vi "DigitalIORead.vi"(0 "error in":errorcluster, 2 "Component":T1, 3 "node":string) -> (1 "error out":errorcluster, 4 "Digital IO State":cluster{"state":i8, "is input only":bool})   [LabVIEW 2015]
doc: "Read a digital output"
uses:
  ROS/Code/SubVIs/DigitalIOComponents.ctl
  ROS/Code/Console/Servers/ServerSubs/TopicDef.ctl
  ROS/Code/SubVIs/_ROSDirection.ctl
panel:
  out "Reply":string
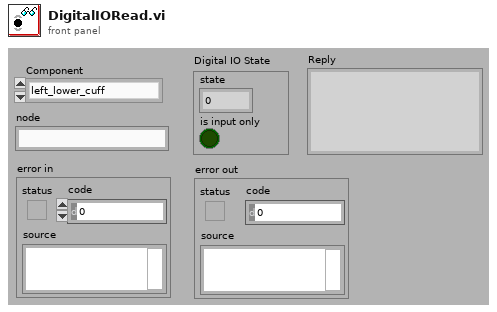
[diagram p1: front panel]
types:
  T1 = typedef "DigitalIOComponents.ctl" = enum16{"left_lower_cuff", "right_lower_cuff", "left_lower_button", "right_lower_button", "left_upper_button", "right_upper_button", "left_shoulder_button", "right_shoulder_button"}
  T2 = typedef "TopicDef.ctl" = cluster{"Topic":string, "Type":string, "Action":T3, "Update (ms)":u16, "queue size":u16}
  T3 = typedef "_ROSDirection.ctl" = enum16{"Node", "Publisher", "Subscriber", "ServiceClient", "ServiceProvider"}
  T4 = typedef "_ROSControl.ctl" = cluster{"topic port":u16, "Node":string, "topic":string, "type":string, "node port":u16, "error ":errorcluster, "Direction":T3, "Update (ms)":u16, "FIFO size":u16}
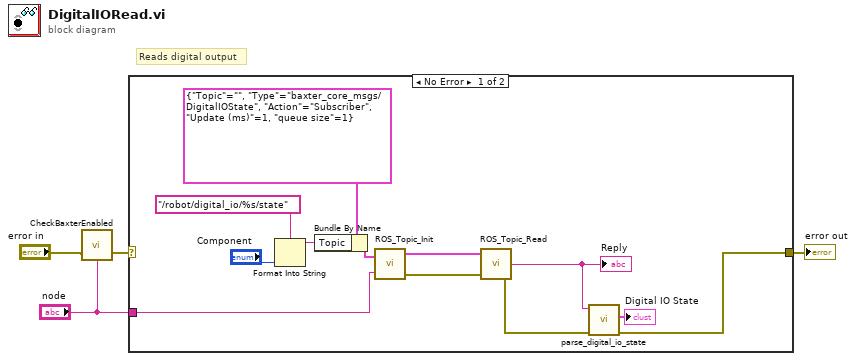
[diagram p0: block diagram]
diagram:
  # "Reads digital output"
  n1 = call "CheckBaxterEnabled.vi"("error in"="error in", "node"="node") -> ("error out"=w2:errorcluster)  [unwired: 2 in]
  n2 = case shown="No Error" w2 {
    selector: w2 -> [_ w17]
    tunnel: [w5 w17] -> w4
    tunnel: "node" -> [w8 _]
    frame No Error {
      n3 = Format Into String(format string="/robot/digital_io/%s/state" ("topic"), "Component") -> (resulting string=w11:string)  [unwired: 2 in, 1 out]
      n4 = Bundle By Name(cluster=T2 {"Topic"="", "Type"="baxter_core_msgs/DigitalIOState", "Action"=enum."Subscriber", "Update (ms)"=1, "queue size"=1} ("Definitions"), "Topic"=w11) -> (w10:T2)
      n5 = call "ROS_Topic_Init.vi"("Definitions"=w10, "node"=w8) -> ("ROS out"=w16:T4, "error out"=w6:errorcluster)  [unwired: 1 in]
      n6 = call "ROS_Topic_Read.vi"("error in (no error)"=w6, "ROS in"=w16) -> ("error out"=w7:errorcluster, "Reply"=w15:string)  [unwired: 1 in, 1 out]
      "Reply" <- w15
      n7 = call "parse_digital_io_state.vi"("error in"=w7, "msg in"=w15) -> ("error out"=w5:errorcluster, "Digital IO State"=→"Digital IO State":cluster{"state":i8, "is input only":bool})  [unwired: 3 in, 1 out]
    }
    frame Error {
    }
  }
  "error out" <- w4
